vi "Error Message Data to String.vi"(8 "error in (no error)":errorcluster, 10 "Error Message Data":T1, 11 "Text Log In":refnum<class "Text Log.lvclass">) -> (0 "error out":errorcluster, 3 "Text Log Out":refnum<class "Text Log.lvclass">)   [LabVIEW 2020, in "Error Log Classes.lvlib" / "Text Log.lvclass"]
uses:
  Text Log.lvclass
  Process Classes/Error Handler/Public/TypeDefs/Error Message Data.ctl
  Text Log.lvclass/Text Log.ctl
  Process Classes/Error Handler/Error Handler.lvclass
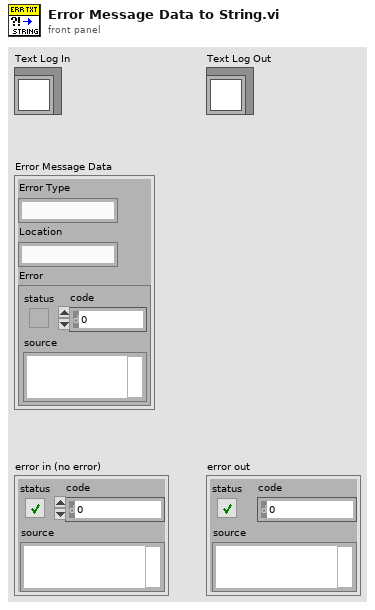
[diagram p1: front panel]
types:
  T1 = typedef "Error Handler.lvclass/Error Message Data.ctl" = cluster{"Error Type":string, "Location":string, "Error":errorcluster}
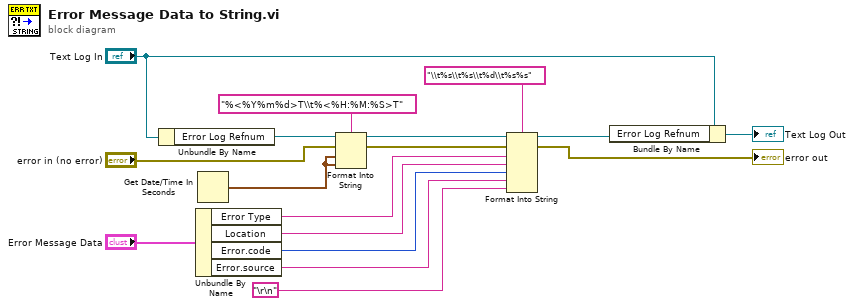
[diagram p0: block diagram]
diagram:
  n1 = Unbundle By Name("Text Log In") -> ("Error Log Refnum"=w15:refnum<file>)
  n2 = Unbundle By Name("Error Message Data") -> ("Error Type"=w13:string, "Location"=w12:string, "Error.code"=w11:i32, "Error.source"=w10:string)
  n3 = Get Date/Time In Seconds() -> (seconds since 1Jan1904=w3:timestamp)
  n4 = Format Into String(format string="%<%Y%m%d>T\\t%<%H:%M:%S>T", initial string=w15, error in="error in (no error)", w3, w3) -> (resulting string=w6:refnum<file>, error out=w5:errorcluster)
  n5 = Format Into String(format string="\\t%s\\t%s\\t%d\\t%s%s", initial string=w6, error in=w5, w13, w12, w11, w10, "\r\n") -> (resulting string=w16:refnum<file>, error out=→"error out":errorcluster)
  n6 = Bundle By Name(cluster="Text Log In", "Error Log Refnum"=w16) -> (→"Text Log Out":refnum<class "Text Log.lvclass">)
